vi "communicatorManager.vi"(8 "error in (no error)":errorcluster, 11 "TCPServer in":refnum<class "TCPServer.lvclass">) -> (0 "error out":errorcluster, 3 "TCPServer out":refnum<class "TCPServer.lvclass">)   [LabVIEW 2016, in "TCPServer.lvclass"]
uses:
  TCPServer.lvclass
panel:
  out "String":string
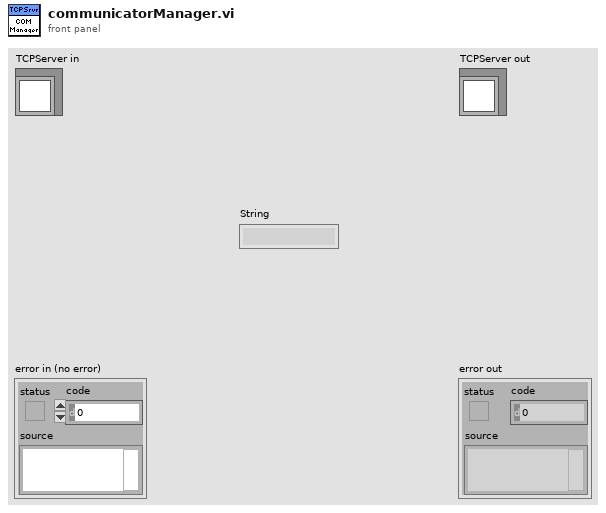
[diagram p1: front panel]
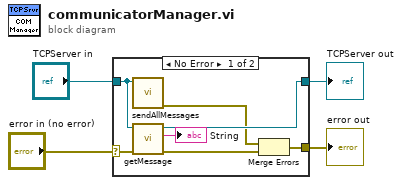
[diagram p0: block diagram]
diagram:
  n1 = case shown="No Error" "error in (no error)" {
    selector: "error in (no error)" -> [w9 w13]
    tunnel: [w8 w13] -> w4
    tunnel: [w10 w12] -> w2
    tunnel: "TCPServer in" -> [w11 w12]
    frame No Error {
      n2 = call "sendAllMessages.vi"("TCPServer in"=w11) -> ("error out"=w7:errorcluster)  [unwired: 9 in, 1 out]
      n3 = call-dynamic "getMessage.vi"("error in (no error)"=w9, "TCPServer in"=w11) -> ("error out"=w6:errorcluster, "String"=→"String":string, "TCPServer out"=w10:refnum<class "TCPServer.lvclass">)  [unwired: 7 in]
      n4 = Merge Errors(w7, w6) -> (w8:errorcluster)
    }
    frame Error {
    }
  }
  "error out" <- w4
  "TCPServer out" <- w2
